vi "Selec_COM.vi"(11 "UI Data IN":T1) -> (3 "UI Data OUT":T1)   [LabVIEW 2019]
uses:
  6 SEMESTRE/MICROPROCESADORES_AVANZADOS/P5_P2/INTERFACE_LABVIEW/INTERFACE UI Data.ctl
panel:
  in  "SELECCIONAR COM":refnum<visa-resource-name>
  in  "Aceptar":bool
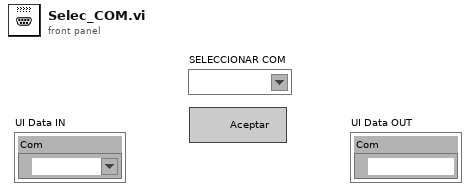
[diagram p1: front panel]
types:
  T1 = typedef "INTERFACE UI Data.ctl" = cluster{"Com":refnum<visa-resource-name>}
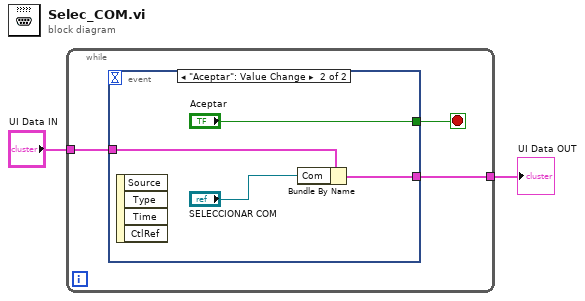
[diagram p0: block diagram]
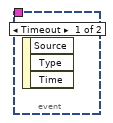
[diagram p2: hidden frame]
diagram:
  n1 = while {
    tunnel: "UI Data IN" -> [w5]
    tunnel: [w3] -> w1
    stop <- w4 stop-if-true
    n2 = event shown="[1] \"Aceptar\": Value Change" {
      selector: _ -> [_ _]
      dyn-events: _ -> [_ _]
      timeout: _ -> [_ _]
      tunnel: w5 -> [_ w9]
      tunnel: [_ "Aceptar"] -> w4
      tunnel: [_ w6] -> w3
      event Timeout {
        n3 = event-data() -> ()  [unwired: 1 in, 3 out]
      }
      event "Aceptar": Value Change {
        n4 = event-data() -> ()  [unwired: 1 in, 4 out]
        n5 = Bundle By Name(cluster=w9, "Com"="SELECCIONAR COM") -> (w6:T1)
      }
    }
  }
  "UI Data OUT" <- w1
